vi "Get received proceed.vi"(8 "error in (no error)":errorcluster, 11 "Autofocus in":refnum<class "Autofocus.lvclass">) -> (0 "error out":errorcluster, 1 "received proceed from camera?":bool, 2 "received proceed from stage?":bool, 3 "Autofocus out":refnum<class "Autofocus.lvclass">)   [LabVIEW 2012, in "Autofocus.lvclass"]
uses:
  Autofocus.lvclass
  Autofocus.lvclass/Autofocus.ctl
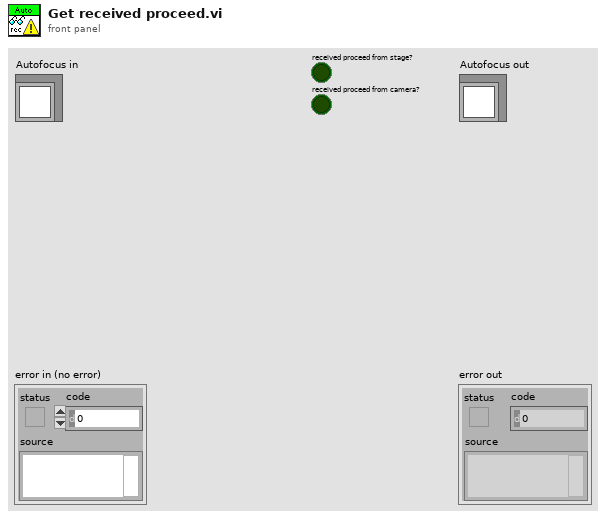
[diagram p1: front panel]
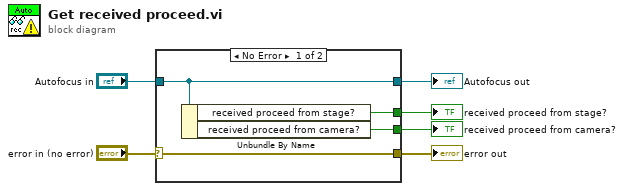
[diagram p0: block diagram]
diagram:
  n1 = case shown="No Error" "error in (no error)" {
    selector: "error in (no error)" -> [w10 w12]
    tunnel: [w10 w12] -> w5
    tunnel: [w9 w11] -> w3
    tunnel: "Autofocus in" -> [w9 w11]
    tunnel: [w8 _] -> w2
    tunnel: [w7 _] -> w1
    frame No Error {
      n2 = Unbundle By Name(w9) -> ("received proceed from stage?"=w8:bool, "received proceed from camera?"=w7:bool)
    }
    frame Error {
    }
  }
  "error out" <- w5
  "Autofocus out" <- w3
  "received proceed from stage?" <- w2
  "received proceed from camera?" <- w1
